vi "Read String.vi"(7 "Channel Index":i32, 8 "error in (no error)":errorcluster, 11 "CIFCorePlugin in":refnum<class "CIFCorePlugin.lvclass">) -> (0 "error out":errorcluster, 2 "Data":string, 3 "CIFCorePlugin out":refnum<class "CIFCorePlugin.lvclass">)   [LabVIEW 2021, in "CIFCorePlugin.lvclass"]
uses:
  CIFCorePlugin.lvclass
  CIFCorePlugin.lvclass/CIFCorePlugin.ctl
  <vilib>/CIF Foundation/CIF Channels Core/CIFChannels/CIFChannels.lvclass
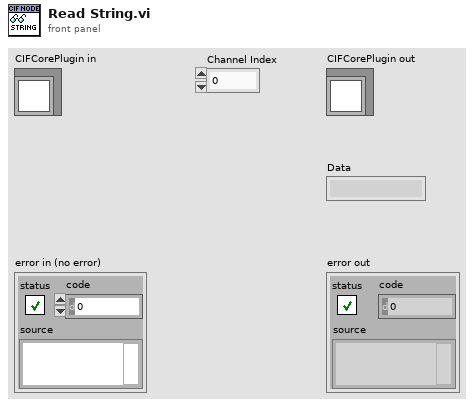
[diagram p1: front panel]
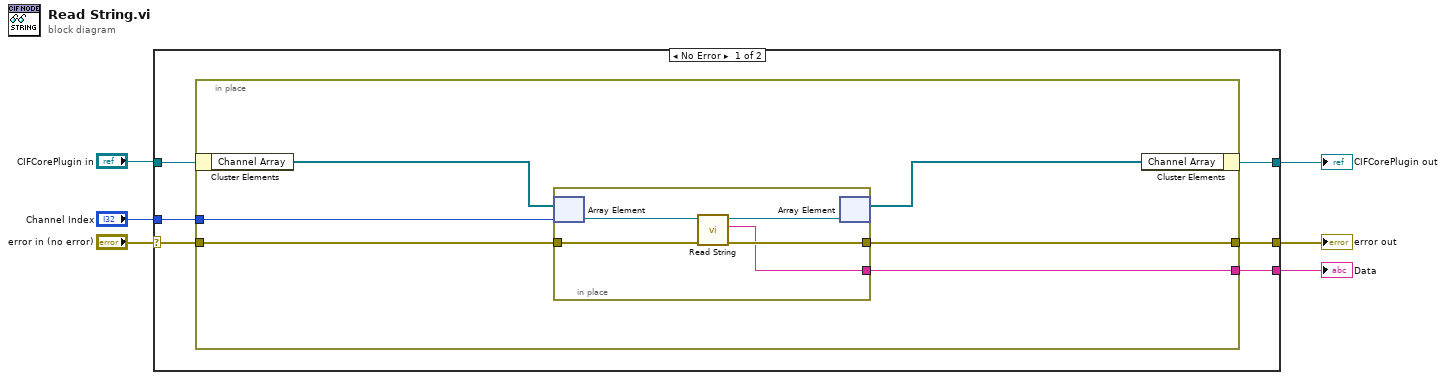
[diagram p0: block diagram]
diagram:
  n1 = case shown="No Error" "error in (no error)" {
    selector: "error in (no error)" -> [w12 w25]
    tunnel: [w11 w25] -> w3
    tunnel: [w8 w24] -> w4
    tunnel: "CIFCorePlugin in" -> [w9 w24]
    tunnel: [w10 _] -> w5
    tunnel: "Channel Index" -> [w7 _]
    frame No Error {
      n2 = in-place {
        in-place-border: w12 -> [w13]
        in-place-border: [w14] -> w11
        in-place-border: [w18] -> w10
        in-place-border: w7 -> [w17]
        n3 = in-place-cluster #1(w9) -> ("Channel Array"=w16:refnum<class "CIFChannels.lvclass">[])
        n4 = in-place {
          in-place-border: w13 -> [w23]
          in-place-border: [w21] -> w14
          in-place-border: [w19] -> w18
          n5 = in-place-array #2(w16, w17) -> (w22:refnum<class "CIFChannels.lvclass">)
          n6 = call-dynamic "Read String.vi"("error in (no error)"=w23, "CIFChannels in"=w22) -> ("error out"=w21:errorcluster, "Data"=w19:string, "CIFChannels out"=w20:refnum<class "CIFChannels.lvclass">)  [unwired: 6 in, 1 out]
          n7 = in-place-array #2(w20) -> (w15:refnum<class "CIFChannels.lvclass">[])  [unwired: 1 out]
        }
        n8 = in-place-cluster #1("Channel Array"=w15) -> (w8:refnum<class "CIFCorePlugin.lvclass">)
      }
    }
    frame Error {
    }
  }
  "error out" <- w3
  "CIFCorePlugin out" <- w4
  "Data" <- w5
